vi "servidor_teste.vi"() -> ()   [LabVIEW 2013]
panel:
  out "String":string
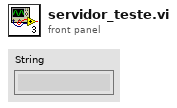
[diagram p1: front panel]
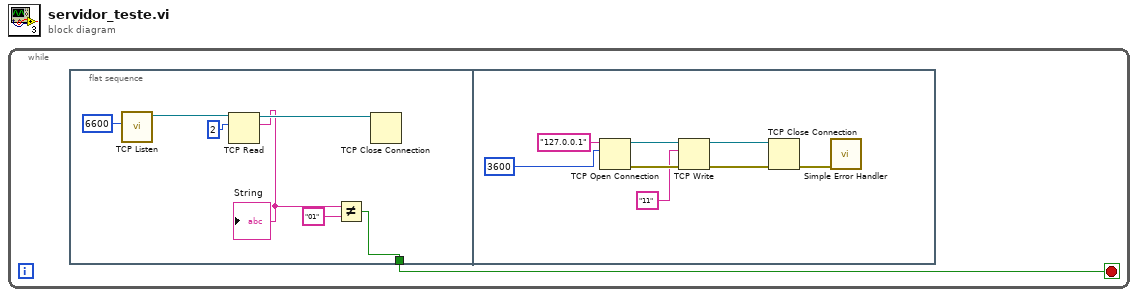
[diagram p0: block diagram]
diagram:
  n1 = while {
    stop <- w1 stop-if-true
    n2 = flat-sequence {
      tunnel: [w2] -> w1
      frame #0 {
        n3 = call <vilib>:"TCP Listen.vi"("port"=u16 6600) -> ("connection ID"=w6:refnum<k5>)  [unwired: 6 in, 4 out]
        n4 = TCP Read(connection ID=w6, bytes to read=2) -> (connection ID out=w8:refnum<k5>, data out=w4:string)  [unwired: 3 in, 1 out]
        "String" <- w4
        n5 = Not Equal?(x=w4, y="01") -> (x != y?=w2:bool)
        n6 = TCP Close Connection(connection ID=w8) -> ()  [unwired: 2 in, 2 out]
      }
      frame #1 {
        n7 = TCP Open Connection(address="127.0.0.1", remote port or service name=u16 3600) -> (connection ID=w16:refnum<k5>, error out=w15:errorcluster)  [unwired: 3 in]
        n8 = TCP Write(connection ID=w16, data in="11", error in (no error)=w15) -> (connection ID out=w14:refnum<k5>, error out=w13:errorcluster)  [unwired: 1 in, 1 out]
        n9 = TCP Close Connection(connection ID=w14, error in (no error)=w13) -> (error out=w12:errorcluster)  [unwired: 1 in, 1 out]
        n10 = call <vilib>:"Simple Error Handler.vi"("error in (no error)"=w12) -> ()  [unwired: 4 in, 5 out]
      }
    }
  }
